vi "Go_to_Idle.vi"(8 "error in (no error)":errorcluster, 11 "Display_Console in":refnum<class "Display_Console.lvclass">) -> (0 "error out":errorcluster, 3 "State out":refnum<class "State Actor.lvclass">)   [LabVIEW 2025, in "Display_Console.lvlib" / "Display_Console.lvclass"]
uses:
  Display_Console.lvclass
  Display_Console.lvclass/Display_Console.ctl
  C:/Program Files (x86)/National Instruments/LabVIEW 2025/vi.lib/ni/Actors/State Actor/State Actor/State Actor.lvclass
  C:/Program Files (x86)/National Instruments/LabVIEW 2025/vi.lib/ActorFramework/Actor/Actor.lvclass
  C:/Users/halstead_rideriver/Documents/Labview_Practice/ATM_Machine_Actor Framework/ATM_ACTORFW/Display_Console/Display_Console/Display_Console.lvclass
  DC_Idle/DC_Idle.lvclass
  C:/Users/halstead_rideriver/Documents/Labview_Practice/ATM_Machine_Actor Framework/ATM_ACTORFW/Display_Console/DC_Idle/DC_Idle.lvclass
  <vilib>/ni/Actors/State Actor/State Actor/State Actor.lvclass
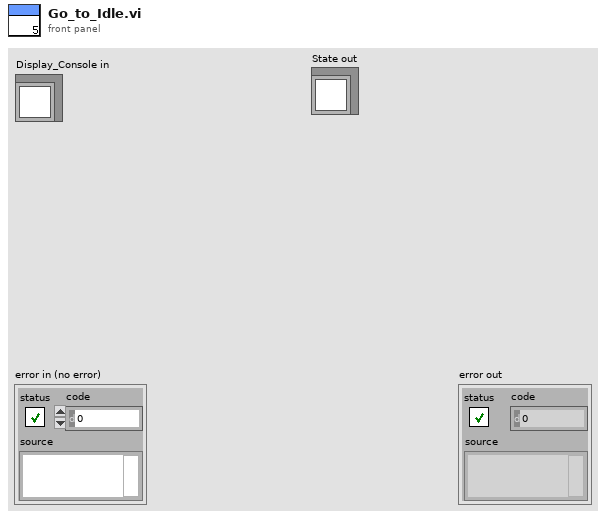
[diagram p1: front panel]
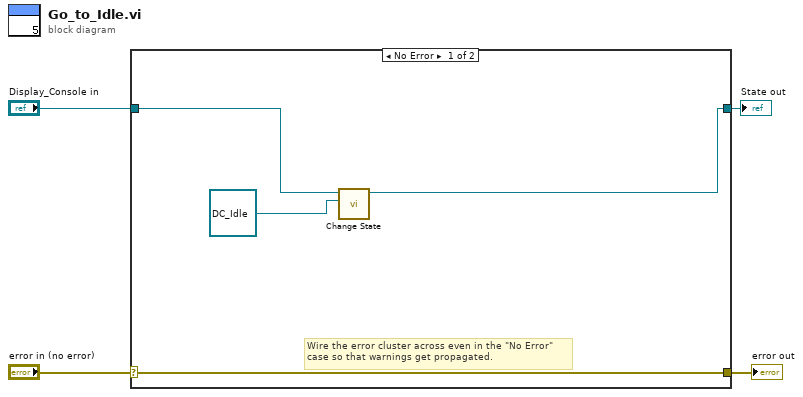
[diagram p0: block diagram]
diagram:
  n1 = case shown="No Error" "error in (no error)" {
    selector: "error in (no error)" -> [w8 w10]
    tunnel: [w8 w10] -> w3
    tunnel: [w5 w9] -> w1
    tunnel: "Display_Console in" -> [w7 w9]
    frame No Error {
      # "Wire the error cluster across even in the \"No Error\"\ncase so that warnings get propagated."
      n2 = call <vilib>:"Change State.vi"("New State in"=refnum<class "DC_Idle.lvclass"> refnum ("Display_Console.lvlib:DC_Idle.lvclass"), "State in"=w7) -> ("State out"=w5:refnum<class "State Actor.lvclass">)  [unwired: 8 in, 1 out]
    }
    frame Error {
    }
  }
  "error out" <- w3
  "State out" <- w1
